vi "Get Master-Slave Relationship.vi"(4 "error in (no error)":errorcluster, 6 "Slave Axis":i32=1 min=1 max=3, 7 "VISA resource name":refnum<visa-resource-name>) -> (0 "error out":errorcluster, 2 "Master Axis":i32, 3 "VISA resource name out":refnum<visa-resource-name>)   [LabVIEW 2020, in "Newport ESP301.lvlib"]
doc: "query the master axis number for slave axis."
uses:
  Newport ESP301.lvlib
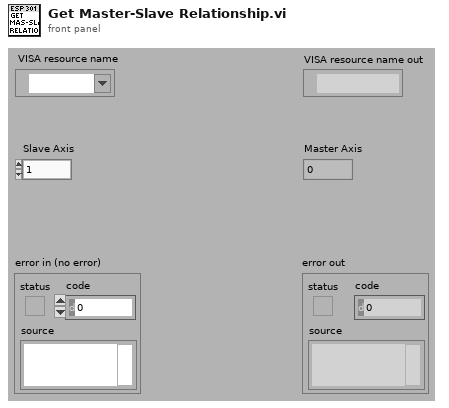
[diagram p1: front panel]
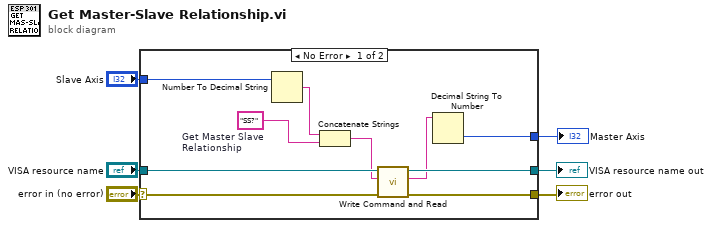
[diagram p0: block diagram]
diagram:
  n1 = case shown="No Error" "error in (no error)" {
    selector: "error in (no error)" -> [w15 w18]
    tunnel: [w14 w18] -> w5
    tunnel: "VISA resource name" -> [w16 w17]
    tunnel: [w13 w17] -> w3
    tunnel: "Slave Axis" -> [w10 _]
    tunnel: [w7 _] -> w1
    frame No Error {
      w12 = "SS?"  # Get Master Slave  Relationship
      n2 = Number To Decimal String(number=w10) -> (decimal integer string=w11:string)  [unwired: 1 in]
      n3 = Concatenate Strings(w11, w12) -> (w9:string)
      n4 = call "Write Command and Read.vi"("error in (no error)"=w15, "Command"=w9, "VISA resource name"=w16) -> ("error out"=w14:errorcluster, "Returned string"=w8:string, "VISA resource name out"=w13:refnum<visa-resource-name>)  [unwired: 4 in]
      n5 = Decimal String To Number(string=w8) -> (number=w7:i32)  [unwired: 2 in, 1 out]
    }
    frame Error {
    }
  }
  "error out" <- w5
  "VISA resource name out" <- w3
  "Master Axis" <- w1
